vi "test-trajectory-generator-01.vi"() -> (3 "Okay":bool)   [LabVIEW 2019]
uses:
  <vilib>/Rock Robotics/WPI/ThirdParty/JAS_Junk/TrajLib/Trajectory_Library.lvlib
panel:
  out "XY Graph 2":cluster{dbl[], dbl[]}[](graph)
  out "XY Graph":cluster{dbl[], dbl[]}(graph)
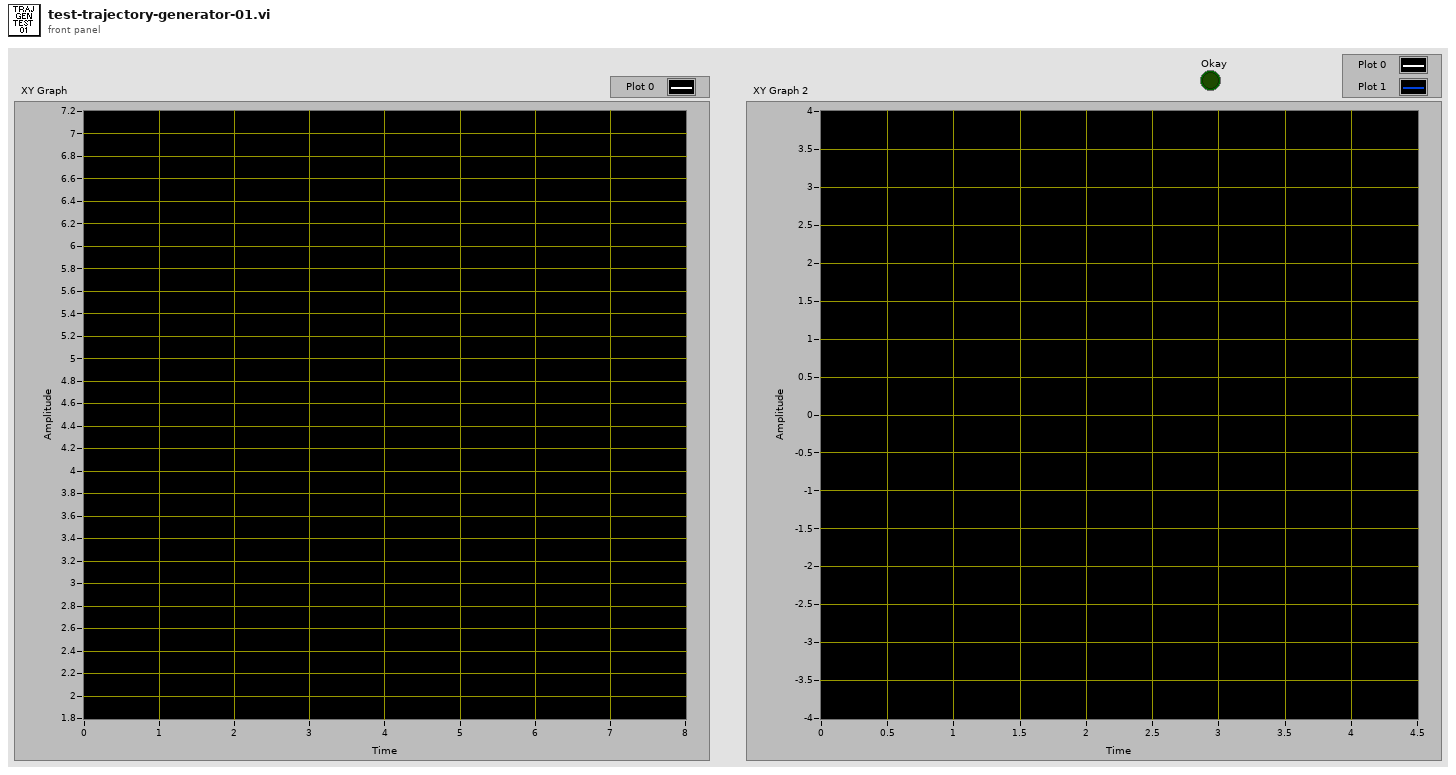
[diagram p1: front panel]
types:
  T1 = typedef "Trajectory_Library.lvlib/TRAJ_CONFIG.ctl" = cluster{"MaxVelocity":dbl, "Max Acceleration":dbl, "StartVelocity":dbl, "End Velocity":dbl, "Reversed":bool, "DiffDrKineConstntDefined":bool, "CentAcellConstntDefined":bool, "DiffDrVoltConstntDefined":bool, "DIFF_DRIVE_KINE_CONSTRAINT":T2, "CENTRIPETAL_ACCEL_CONSTRAINT":T4, "SwerveDrKineConstntDefined":bool, "SWERVE_DRIVE_KINE_CONSTRAINT":T5, "DIFF_DRIVE_VOLTAGE_CONSTRAINT":T9, "MECANUM_DRIVE_KINE_CONSTRAINT":T11, "MecanumDrKineConstntDefined":bool}
  T2 = typedef "Trajectory_Library.lvlib/TRAJ_CONSTRAINT_DIIF_DRIVE_KINEMATICS.ctl" = cluster{"Max Speed (M/S)":dbl, "DIFF_DRIVE_KINEMATICS":T3, "Max Accel (M/S2)":dbl}
  T3 = typedef "Trajectory_Library.lvlib/DIFF_DRIVE_KINEMATICS.ctl" = cluster{"TrackWidth_Meters":dbl}
  T4 = typedef "Trajectory_Library.lvlib/TRAJ_CONSTRAINT_CENTRIPETAL_ACCEL.ctl" = cluster{"Max Cent Accel":dbl}
  T5 = typedef "Trajectory_Library.lvlib/TRAJ_CONSTRAINT_SWERVE_DRIVE_KINEMATICS.ctl" = cluster{"Max Speed (M/S)":dbl, "SwerveKinematics":T6}
  T6 = typedef "Trajectory_Library.lvlib/SWERVE_DRIVE_KINEMATICS.ctl" = cluster{"NumModules":i32, "InverseKinematics":T7, "ForwardKinematics":T7, "Modules":T8[], "PrevCoR":T8}
  T7 = typedef "NI_Matrix.lvlib/RealMatrix.ctl" = dbl[][]
  T8 = typedef "Trajectory_Library.lvlib/TRANSLATION2D.ctl" = cluster{"X":dbl, "Y":dbl}
  T9 = typedef "Trajectory_Library.lvlib/TRAJ_CONSTRAINT_DIIF_DRIVE_VOLTAGE.ctl" = cluster{"Max Voltage":dbl, "DIFF_DRIVE_KINEMATICS":T3, "SIMPLE_MOTOR_FF":T10}
  T10 = typedef "Trajectory_Library.lvlib/SIMPLE_MOTOR_FF.ctl" = cluster{"Ks":dbl, "Kv":dbl, "Ka":dbl}
  T11 = typedef "Trajectory_Library.lvlib/TRAJ_CONSTRAINT_MECA_DRIVE_KINEMATICS.ctl" = cluster{"Max Speed (M/S)":dbl, "MECA_DRIVE_KINEMATICS":T12}
  T12 = typedef "Trajectory_Library.lvlib/MECA_DRIVE_KINEMATICS.ctl" = cluster{"FrontLeft":T8, "FrontRight":T8, "RearLeft":T8, "RearRight":T8, "InverseKinematics":T7, "ForwardKinematics":T7, "PrevCoR":T8}
  T13 = typedef "Trajectory_Library.lvlib/TRAJECTORY.ctl" = cluster{"TotalTImeSecs":dbl, "States":T14[]}
  T14 = typedef "Trajectory_Library.lvlib/TRAJ_STATE.ctl" = cluster{"TimeSeconds":dbl, "Velocity":dbl, "Acceleration":dbl, "POSE":T15, "Curvature":dbl}
  T15 = typedef "Trajectory_Library.lvlib/POSE2D.ctl" = cluster{"TRANSLATION":T8, "ROTATION":T16}
  T16 = typedef "Trajectory_Library.lvlib/ROTATION2D.ctl" = cluster{"VALUE":dbl, "COS":dbl, "SIN":dbl}
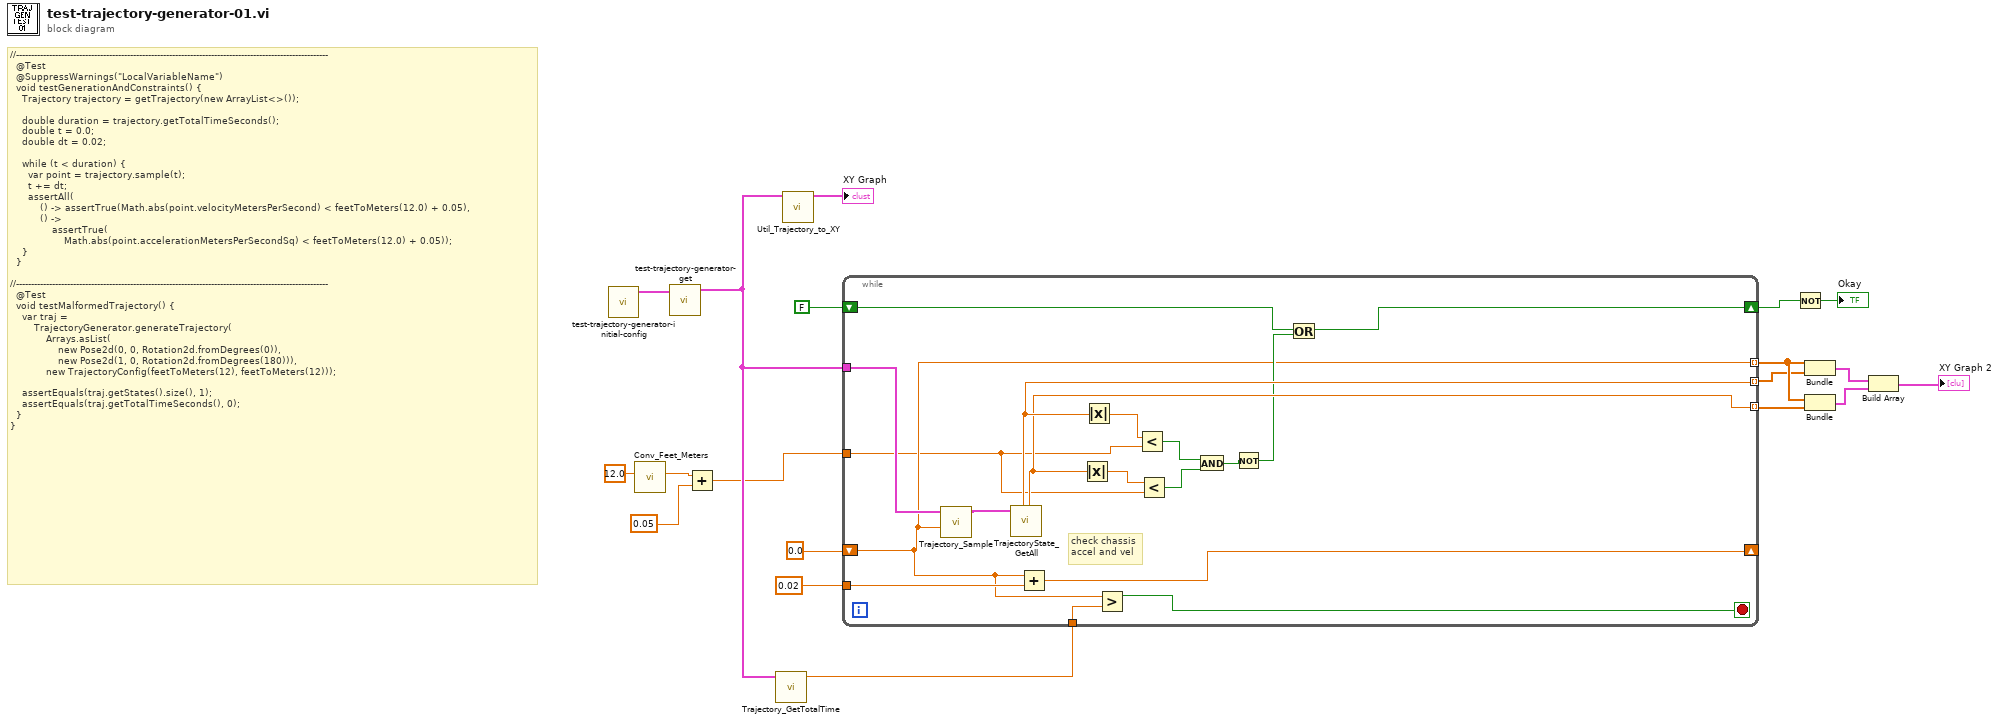
[diagram p0: block diagram]
diagram:
  # "//--------------------------------------------------------------------------------------------------------\n  @Test\n  @SuppressWarnings(\"LocalVariableName\")\n  void testGenerationAndConstraints() {\n    Trajectory trajectory = getTrajectory(new ArrayList<>());\n\n    double duration = trajectory.getTotalTimeSeconds();\n    double t = 0.0;\n    double dt = 0.02;\n\n    while (t < duration) {\n      var point = trajectory.sample(t);\n      t += dt;\n      assertAll(\n          () -> assertTrue(Math.abs(point.velocityMetersPerSecond) < feetToMeters(12.0) + 0.05),\n          () ->\n              assertTrue(\n                  Math.abs(point.accelerationMetersPerSecondSq) < feetToMeters(12.0) + 0.05));\n    }\n  }\n\n//--------------------------------------------------------------------------------------------------------\n  @Test\n  void testMalformedTrajectory() {\n    var traj =\n        TrajectoryGenerator.generateTrajectory(\n            Arrays.asList(\n                new Pose2d(0, 0, Rotation2d.fromDegrees(0)),\n                new Pose2d(1, 0, Rotation2d.fromDegrees(180))),\n            new TrajectoryConfig(feetToMeters(12), feetToMeters(12)));\n\n    assertEquals(traj.getStates().size(), 1);\n    assertEquals(traj.getTotalTimeSeconds(), 0);\n  }\n}"
  n1 = call "test-trajectory-generator-initial-config.vi"() -> ("traj_config"=w19:T1)  [unwired: 11 in]
  n2 = call <vilib>:"Conv_Feet_Meters.vi"("Feet"=12.0) -> ("Meters"=w3:dbl)  [unwired: 10 in]
  n3 = call "test-trajectory-generator-get.vi"("traj_config"=w19) -> ("TRAJECTORY"=w6:T13)  [unwired: 8 in, 2 out]
  n4 = Add(x=w3, y=0.05) -> (x+y=w1:dbl)
  n5 = call <vilib>:"Trajectory_GetTotalTime.vi"("TRAJECTORY"=w6) -> ("TotalTime_Sec"=w5:dbl)  [unwired: 10 in]
  n6 = call <vilib>:"Util_Trajectory_to_XY.vi"("TRAJECTORY"=w6) -> ("outArrayXY"=→"XY Graph":cluster{dbl[], dbl[]})  [unwired: 10 in]
  n7 = while {
    tunnel: 0.02 -> [w25]
    shift-right: [w24] -> _
    shift-left: 0.0 -> [w23]
    tunnel: w6 -> [w36]
    tunnel: [w32] -> w14 mode=indexing
    tunnel: [w31] -> w13 mode=indexing
    tunnel: [w23] -> w15 mode=indexing
    shift-right: [w26] -> w8
    shift-left: FALSE -> [w26]
    tunnel: w5 -> [w22]
    tunnel: w1 -> [w20]
    stop <- w21 stop-if-true
    # "check chassis\naccel and vel"
    n8 = call <vilib>:"Trajectory_Sample.vi"("Time"=w23, "InputTRAJECTORY"=w36) -> ("OutputTRAJ_STATE"=w35:T14)  [unwired: 9 in]
    n9 = call <vilib>:"TrajectoryState_GetAll.vi"("TRAJ_STATE"=w35) -> ("Acceleration"=w31:dbl, "Velocity"=w32:dbl)  [unwired: 4 in, 5 out]
    n10 = Add(x=w23, y=w25) -> (x+y=w24:dbl)
    n11 = Absolute Value(x=w31) -> (abs(x)=w33:dbl)
    n12 = Absolute Value(x=w32) -> (abs(x)=w34:dbl)
    n13 = Greater?(x=w23, y=w22) -> (0:w21:bool)
    n14 = Less?(x=w34, y=w20) -> (x < y?=w30:bool)
    n15 = Less?(x=w33, y=w20) -> (x < y?=w29:bool)
    n16 = And(x=w30, y=w29) -> (x .and. y?=w28:bool)
    n17 = Not(x=w28) -> (.not. x?=w27:bool)
    n18 = Or(x=w26, y=w27) -> ()  [unwired: 1 out]
  }
  n19 = Not(x=w8) -> (.not. x?=→"Okay":bool)
  n20 = Bundle(w15, w14) -> (w12:cluster{dbl[], dbl[]})  [unwired: 1 in]
  n21 = Bundle(w15, w13) -> (w11:cluster{dbl[], dbl[]})  [unwired: 1 in]
  n22 = Build Array(w12, w11) -> (→"XY Graph 2":cluster{dbl[], dbl[]}[])
